vi "data_pack.vi"(3 "in_data":i16[][](array[numeric]), 4 "refnum_in":refnum<file>) -> (0 "refnum_out":refnum<file>)   [LabVIEW 2013]
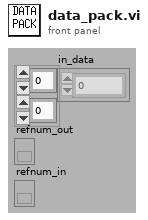
[diagram p1: front panel]
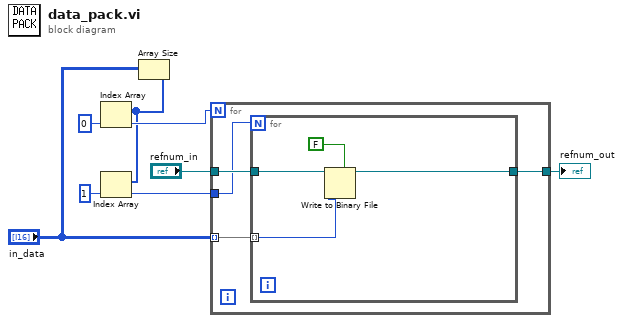
[diagram p0: block diagram]
diagram:
  n1 = Array Size(array="in_data") -> (size(s)=w3:i32[])
  n2 = Index Array(array=w3, index=0) -> (element=w5:i32)
  n3 = Index Array(array=w3, index=1) -> (element=w2:i32)
  n4 = for {
    N: w5 -> [_]
    tunnel: "refnum_in" -> [w12]
    tunnel: [w11] -> w8
    tunnel: "in_data" -> [w10] mode=indexing
    tunnel: w2 -> [w9]
    n5 = for {
      N: w9 -> [_]
      tunnel: w12 -> [w16]
      tunnel: [w15] -> w11
      tunnel: w10 -> [w14] mode=indexing
      n6 = Write to Binary File(file (use dialog)=w16, data=w14, 5:FALSE ("prepend array or string size? (T)")) -> (refnum out=w15:refnum<file>)  [unwired: 3 in, 2 out]
    }
  }
  "refnum_out" <- w8
